vi "DebugInput.vi"(7 "error in (no error)":errorcluster, 9 "Y In":dbl(slide)=50.0 scale=0.0..100.0, 10 "X In":dbl(slide)=50.0 scale=0.0..100.0) -> (0 "error out":errorcluster, 2 "Y Out":dbl(slide) scale=0.0..100.0, 3 "X Out":dbl(slide) scale=0.0..100.0)   [LabVIEW 2016]
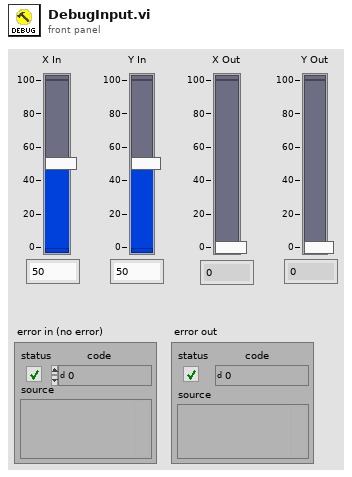
[diagram p1: front panel]
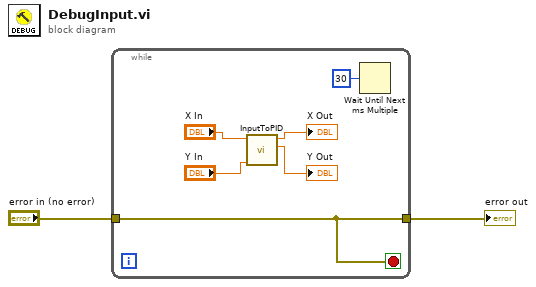
[diagram p0: block diagram]
diagram:
  n1 = while {
    tunnel: [w7] -> w2
    tunnel: "error in (no error)" -> [w7]
    stop <- w7 stop-if-true
    n2 = call "InputToPID.vi"("Y Position In"="Y In", "X Position In"="X In") -> ("Y Position"=→"Y Out":dbl, "X Position"=→"X Out":dbl)  [unwired: 8 in]
    n3 = Wait Until Next ms Multiple(millisecond multiple=u32 30) -> ()  [unwired: 1 out]
  }
  "error out" <- w2
